vi "RFID_28_03_12.vi"(5 "BYTES TO READ":i32, 6 "TIMEOUT":i32, 7 "RFID_Error":errorcluster, 8 "Puerto RFID":u16, 9 "IP RFID":string, 10 "RFID ID":refnum<k5>) -> (0 "RFID Error":errorcluster, 1 "connection ID out":refnum<k5>, 3 "TAGs HEX":string[](array[string]), 4 "Unidad":u32)   [LabVIEW 2015]
panel:
  out "RFID_ID":refnum<k5>
  out "RFID_Error":errorcluster
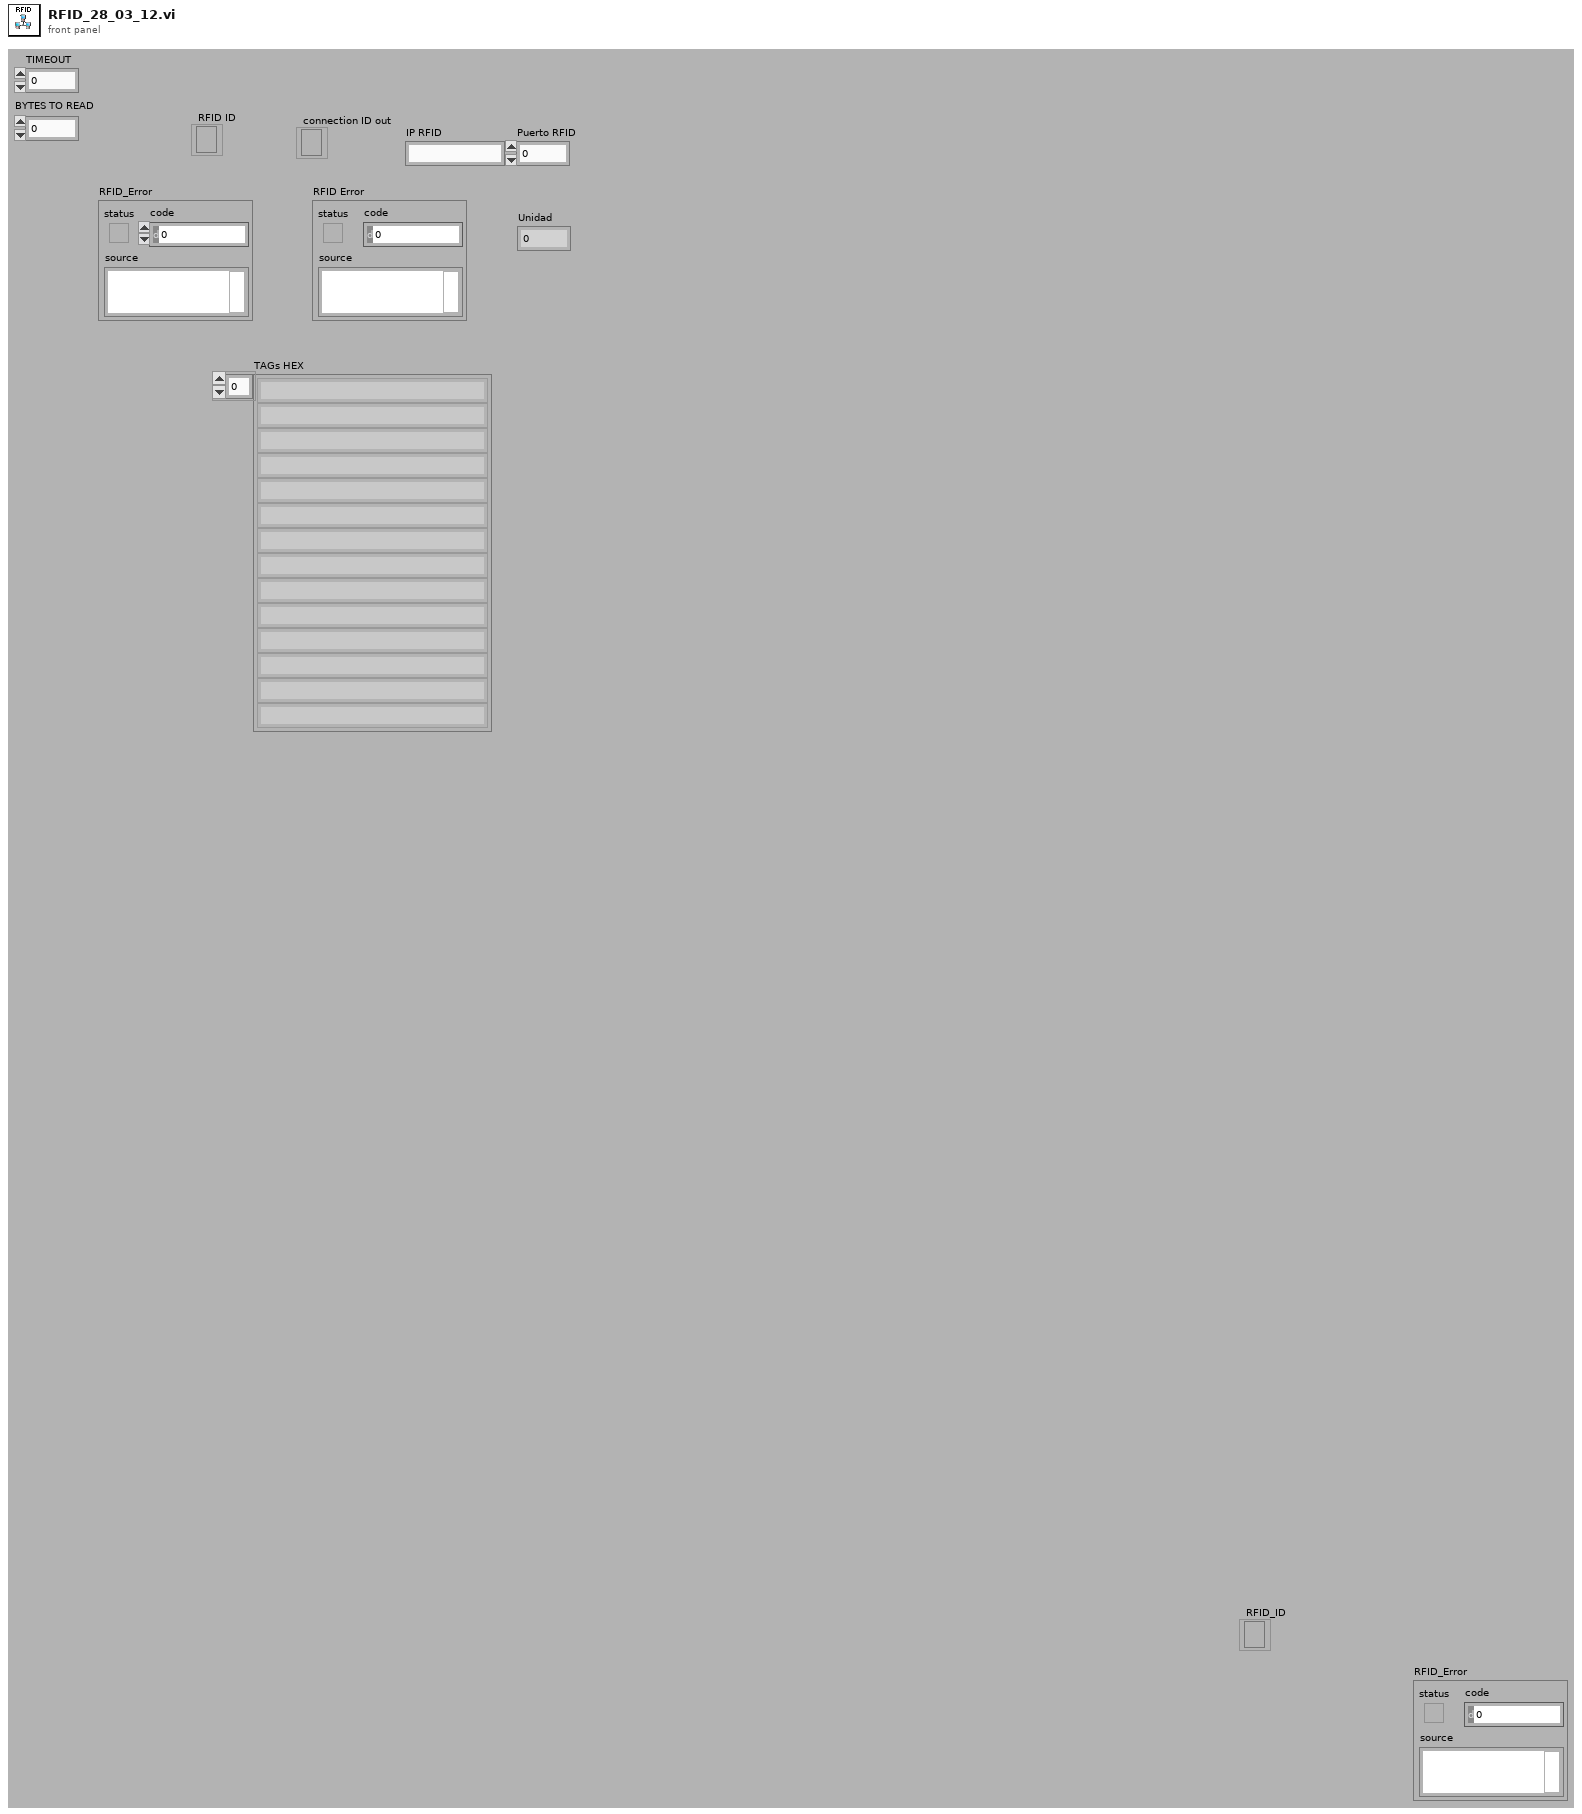
[diagram p1: front panel]
types:
  T1 = enum16{"Standard", "Buffered", "CRLF", "Immediate"}
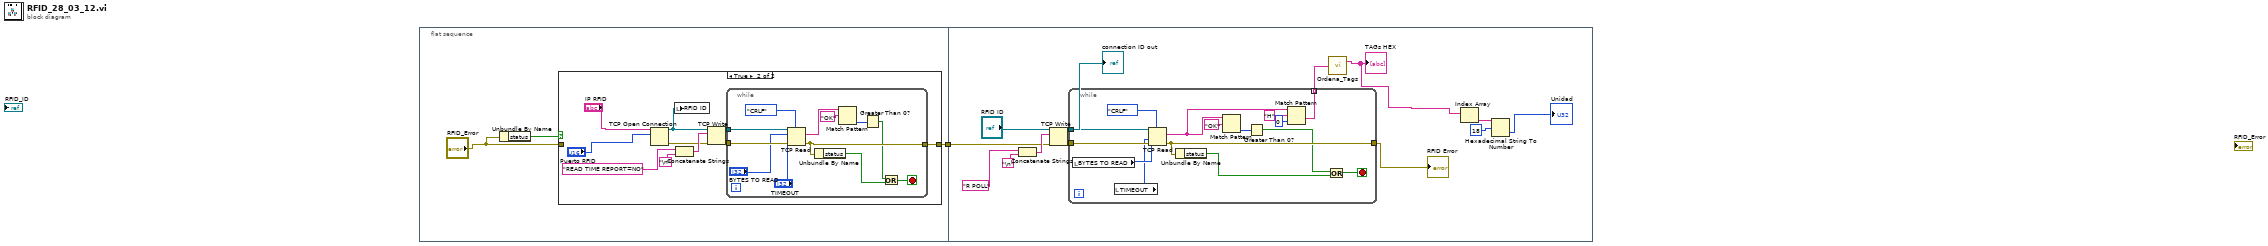
[diagram p0: block diagram]
diagram:
  n1 = flat-sequence {
    tunnel: [w3] -> w1
    tunnel: w1 -> [w34]
    frame #0 {
      n2 = Unbundle By Name("RFID_Error") -> ("status"=w4:bool)
      n3 = case shown="True" w4 {
        tunnel: [w5 w15] -> w3
        tunnel: "RFID_Error" -> [w5 _]
        frame False {
        }
        frame True {
          n4 = TCP Open Connection(address="IP RFID", remote port or service name="Puerto RFID") -> (connection ID=w12:refnum<k5>, error out=w11:errorcluster)  [unwired: 1 in, 2 out]
          n5 = local write "RFID ID"(w12) -> ()
          n6 = Concatenate Strings("READ TIME REPORT=NO" ("data in"), "\n") -> (w13:string)
          n7 = TCP Write(connection ID=w12, data in=w13, error in (no error)=w11) -> (connection ID out=w9:refnum<k5>, error out=w10:errorcluster)  [unwired: 2 out]
          n8 = while {
            tunnel: w10 -> [w26]
            tunnel: w9 -> [w25]
            tunnel: [w24] -> w15
            stop <- w20 stop-if-true
            n9 = TCP Read(connection ID=w25, bytes to read="BYTES TO READ", error in (no error)=w26, 7:T1."CRLF" ("mode (standard)"), 9:"TIMEOUT") -> (data out=w21:string, error out=w24:errorcluster)  [unwired: 1 out]
            n10 = Unbundle By Name(w24) -> ("status"=w19:bool)
            n11 = Match Pattern(string=w21, regular expression="OK") -> (offset past match=w23:i32)  [unwired: 4 out]
            n12 = Greater Than 0?(x=w23) -> (x > 0?=w18:bool)
            n13 = Or(x=w18, y=w19) -> (x .or. y?=w20:bool)
          }
        }
      }
    }
    frame #1 {
      n14 = Concatenate Strings("R POLL" ("string"), "\n") -> (w36:string)
      n15 = TCP Write(connection ID="RFID ID", data in=w36, error in (no error)=w34) -> (connection ID out=w38:refnum<k5>, error out=w37:errorcluster)  [unwired: 1 in, 1 out]
      "connection ID out" <- w38
      n16 = while {
        tunnel: w37 -> [w54]
        tunnel: w38 -> [w53]
        tunnel: [w52] -> w39
        tunnel: [w43] -> w29 mode=indexing
        stop <- w47 stop-if-true
        n17 = local read "BYTES TO READ"() -> (w42:i32)
        n18 = local read "TIMEOUT"() -> (w41:i32)
        n19 = TCP Read(connection ID=w53, bytes to read=w42, error in (no error)=w54, 7:T1."CRLF" ("mode (standard)"), 9:w41) -> (data out=w44:string, error out=w52:errorcluster)  [unwired: 1 out]
        n20 = Unbundle By Name(w52) -> ("status"=w45:bool)
        n21 = Match Pattern(string=w44, regular expression="OK") -> (offset past match=w48:i32)  [unwired: 4 out]
        n22 = Greater Than 0?(x=w48) -> (x > 0?=w46:bool)
        n23 = Match Pattern(string=w44, regular expression="H", offset (0)=0) -> (after substring=w43:string)  [unwired: 3 out]
        n24 = Or(x=w46, y=w45) -> (x .or. y?=w47:bool)
      }
      "RFID Error" <- w39
      n25 = call "Ordena_Tags.vi"("Tags_desorden"=w29) -> ("Array"=w28:string[])  [unwired: 1 out]
      "TAGs HEX" <- w28
      n26 = Index Array(array=w28) -> (element=w31:string)  [unwired: 1 in]
      n27 = Hexadecimal String To Number(string=w31, offset=18) -> (number=→"Unidad":u32)  [unwired: 2 out]
    }
  }
